vi "2012 Host Approach.vi"() -> ()   [LabVIEW 2013]
uses:
  <vilib>/rvi/interface/nirviOpenFPGA/nirviOpenFPGA.xnode
  <vilib>/rvi/interface/nirviReadWriteControl/nirviReadWriteControl.xnode
  <vilib>/rvi/interface/Simulation/niFpgaSimulationCallBeginRW.vi
  <vilib>/rvi/errors/niLvFpgaAdjustHostInterfaceError.vi
  <vilib>/rvi/interface/nirviCloseFPGA/nirviCloseFPGA.xnode
  <vilib>/FPGAPlugInAG/Dynamic/niLvFpga_Close_Dynamic.vi
  <vilib>/rvi/interface/nirviMethod/nirviMethod.xnode
  <vilib>/FPGAPlugInAG/Dynamic/niLvFpga_Run_Dynamic.vi
panel:
  in  "Automated Approach Start":bool
  out "FPGA Output Voltage":dbl(graph)
  in  "MCL Counter":i64
  in  "MCL Divisions":i32
  out "MCL Range Indicator":bool
  out "Host Counter Indicator":i64
  out "Digital Steps per Region":i32
  out "Host Counter Output":i32
  in  "Z Position MCL Fine":i32
  out "Host Z Position Indicator":i32
  out "Z Position Range Indicator":bool
  out "Z Fine Steps per Region":dbl
  out "Host Z Output":fxp<+/-,40,30>
  in  "Manual Approach Start":bool
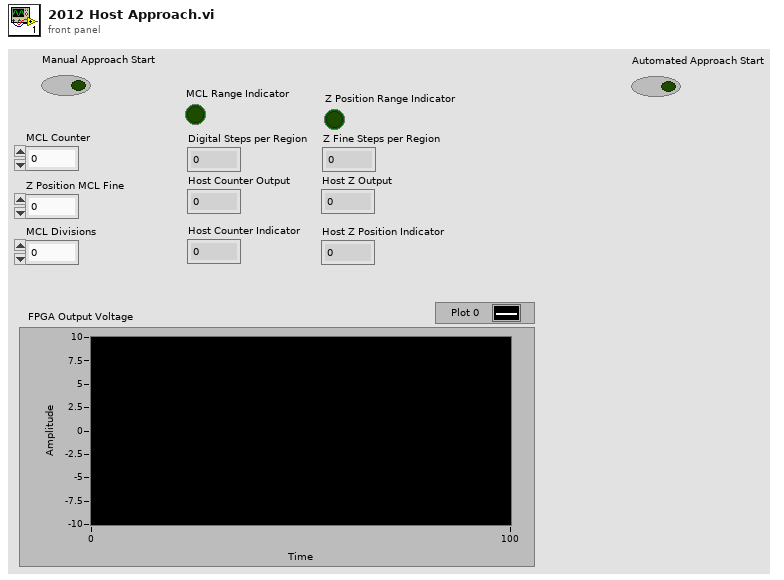
[diagram p1: front panel]
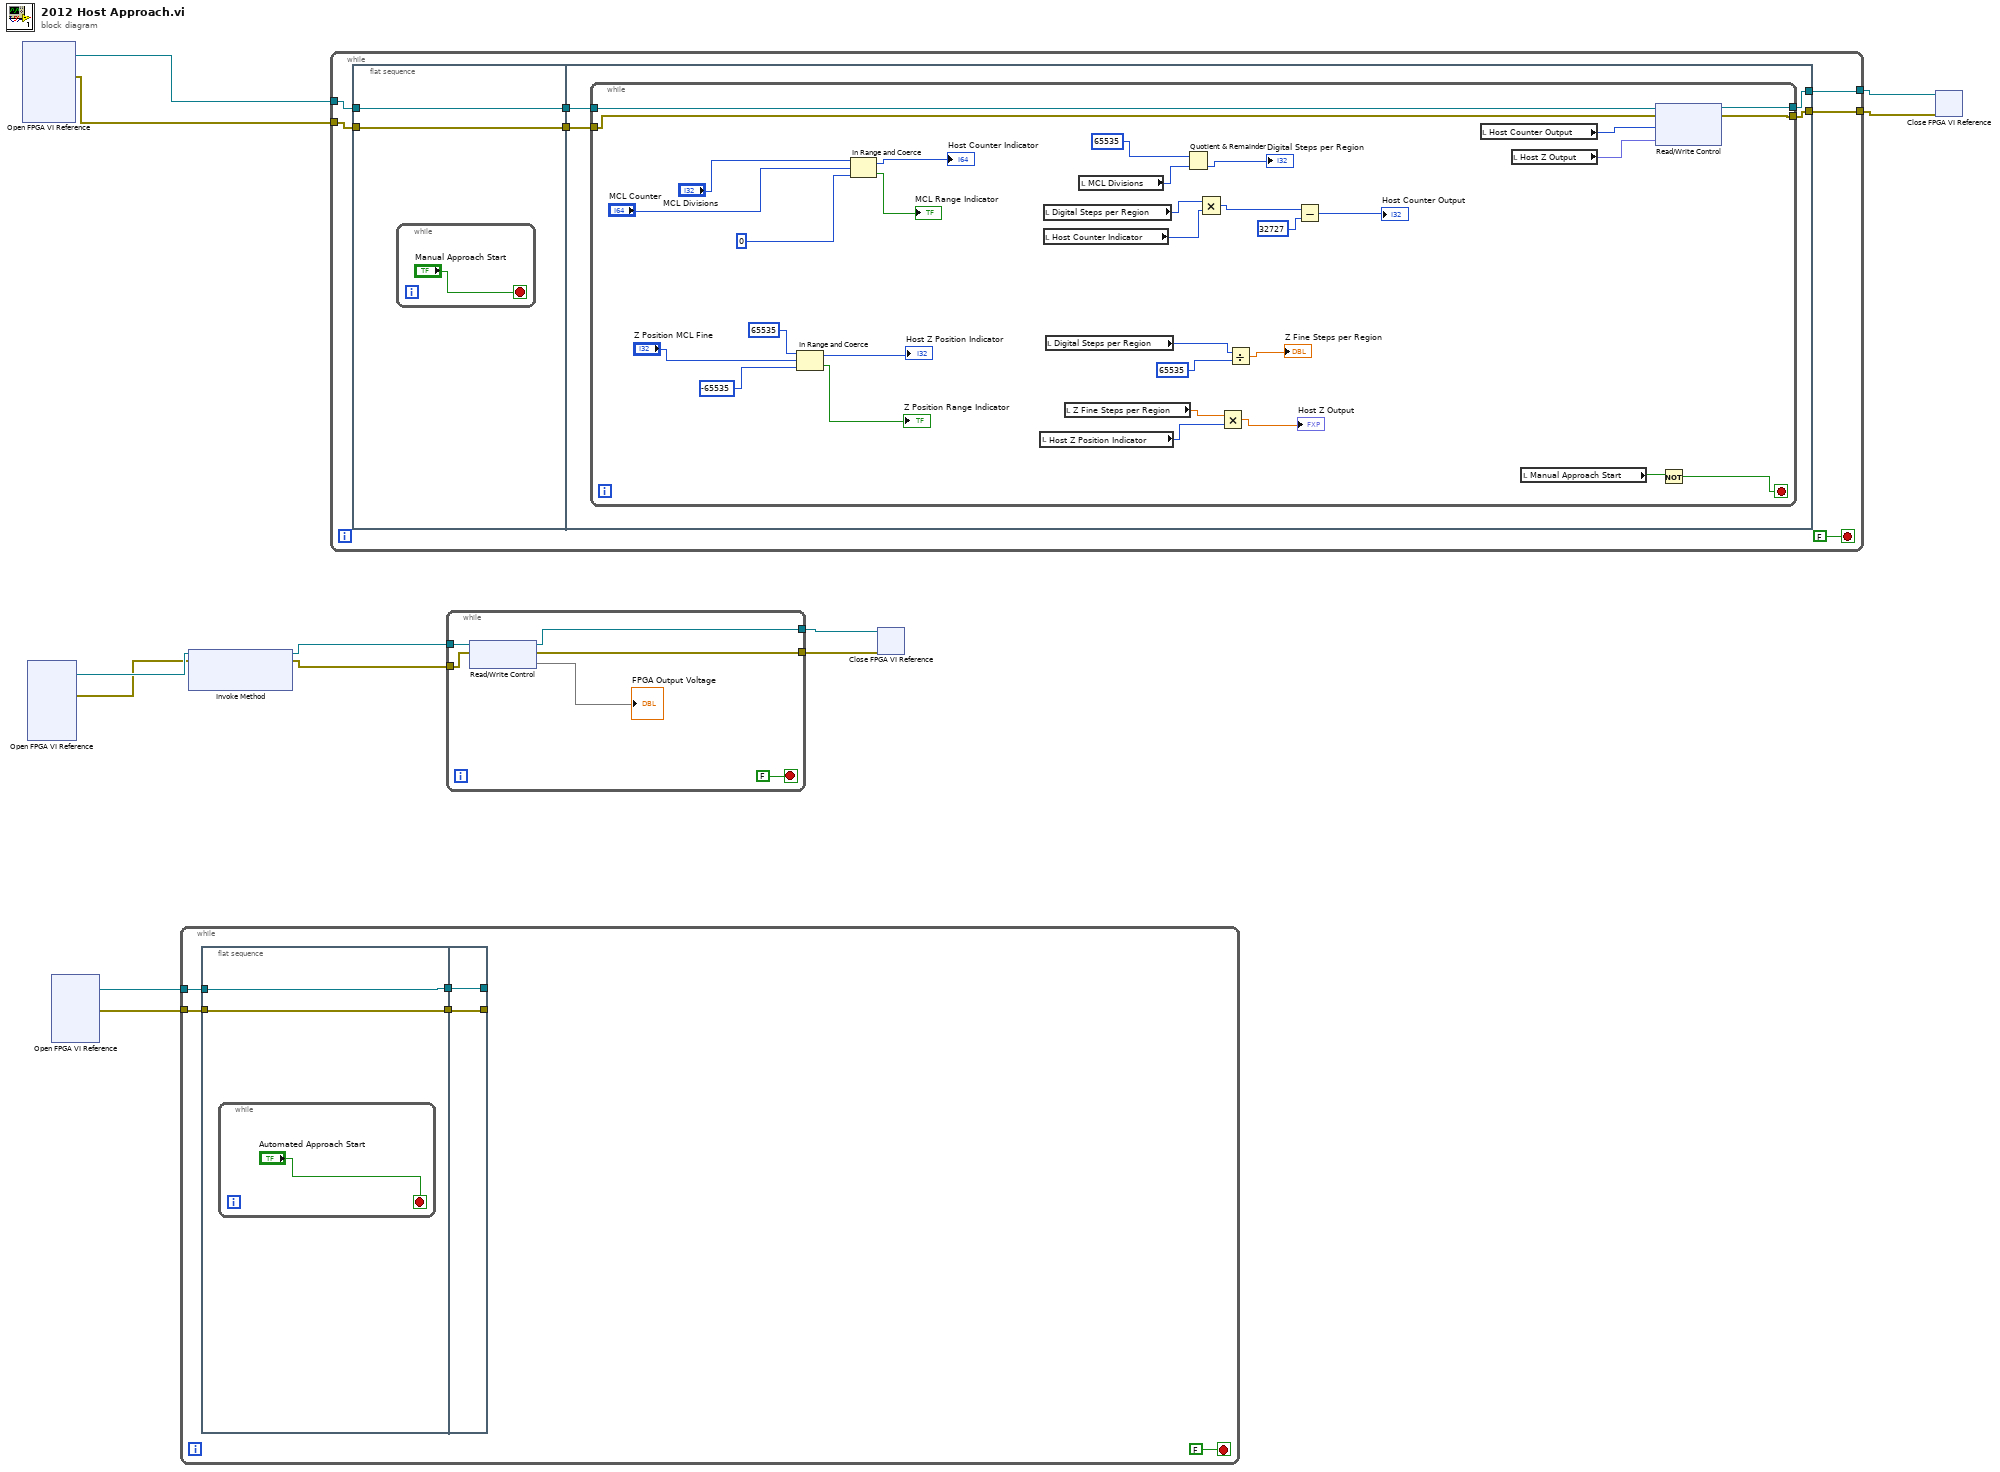
[diagram p0: block diagram]
diagram:
  n1 = xnode "Open FPGA VI Reference"() -> ("FPGA VI Reference Out"=w10:refnum<k20>, "error out"=w9:errorcluster)  [unwired: 2 in]
  n2 = xnode "Open FPGA VI Reference"() -> ("FPGA VI Reference Out"=w4:refnum<k20>, "error out"=w3:errorcluster)  [unwired: 2 in]
  n3 = xnode "Open FPGA VI Reference"() -> ("FPGA VI Reference Out"=w2:refnum<k20>, "error out"=w1:errorcluster)  [unwired: 2 in]
  n4 = while {
    tunnel: w2 -> [w16]
    tunnel: w1 -> [w15]
    stop <- FALSE stop-if-true
    n5 = flat-sequence {
      tunnel: w16 -> [w19]
      tunnel: w15 -> [w18]
      tunnel: [w19] -> w14
      tunnel: [w18] -> w13
      tunnel: [w21] -> _
      tunnel: [w22] -> _
      tunnel: w14 -> [w22]
      tunnel: w13 -> [w21]
      frame #0 {
        n6 = while {
          stop <- "Automated Approach Start" stop-if-true
        }
      }
      frame #1 {
      }
    }
  }
  n7 = xnode "Invoke Method"("FPGA VI Reference In"=w4, "error in"=w3) -> ("FPGA VI Reference Out"=w6:refnum<k20>, "error out"=w5:errorcluster)  [unwired: 1 in]
  n8 = while {
    tunnel: [w28] -> w12
    tunnel: [w27] -> w11
    tunnel: w10 -> [w25]
    tunnel: w9 -> [w23]
    stop <- FALSE stop-if-true
    n9 = flat-sequence {
      tunnel: [w31] -> w26
      tunnel: w25 -> [w31]
      tunnel: [w30] -> w24
      tunnel: w23 -> [w30]
      tunnel: [w34] -> w28
      tunnel: [w33] -> w27
      tunnel: w26 -> [w36]
      tunnel: w24 -> [w35]
      frame #0 {
        n10 = while {
          stop <- "Manual Approach Start" stop-if-true
        }
      }
      frame #1 {
        n11 = while {
          tunnel: w36 -> [w68]
          tunnel: w35 -> [w67]
          tunnel: [w66] -> w34
          tunnel: [w65] -> w33
          stop <- w63 stop-if-true
          n12 = In Range and Coerce(upper limit=65535, x="Z Position MCL Fine", lower limit=-65535) -> (coerced(x)=→"Host Z Position Indicator":i32, In Range?=→"Z Position Range Indicator":bool)
          n13 = In Range and Coerce(upper limit="MCL Divisions", x="MCL Counter", lower limit=0) -> (coerced(x)=→"Host Counter Indicator":i64, In Range?=→"MCL Range Indicator":bool)
          n14 = local read "Host Z Position Indicator"() -> (w39:i32)
          n15 = local read "Digital Steps per Region"() -> (w52:i32)
          n16 = local read "Host Counter Indicator"() -> (w51:i64)
          n17 = local read "Digital Steps per Region"() -> (w43:i32)
          n18 = local read "Z Fine Steps per Region"() -> (w40:dbl)
          n19 = local read "MCL Divisions"() -> (w56:i32)
          n20 = Quotient & Remainder(x=65535, y=w56) -> (floor(x/y)=→"Digital Steps per Region":i32)  [unwired: 1 out]
          n21 = Multiply(x=w52, y=w51) -> (x*y=w53:i64)
          n22 = Multiply(x=w40, y=w39) -> (x*y=→"Host Z Output":dbl)
          n23 = Divide(x=w43, y=65535) -> (x/y=→"Z Fine Steps per Region":dbl)
          n24 = Subtract(x=w53, y=32727) -> (x-y=→"Host Counter Output":i64)
          n25 = local read "Host Counter Output"() -> (w49:i32)
          n26 = local read "Host Z Output"() -> (w37:fxp<+/-,40,30>)
          n27 = local read "Manual Approach Start"() -> (w64:bool)
          n28 = xnode "Read/Write Control"("FPGA VI Reference In"=w68, "error in"=w67, "Unselected"=w49, "Unselected"=w37) -> ("FPGA VI Reference Out"=w66:refnum<k20>, "error out"=w65:errorcluster)
          n29 = Not(x=w64) -> (.not. x?=w63:bool)
        }
      }
    }
  }
  n30 = while {
    tunnel: w6 -> [w73]
    tunnel: w5 -> [w72]
    tunnel: [w71] -> w8
    tunnel: [w70] -> w7
    stop <- FALSE stop-if-true
    n31 = xnode "Read/Write Control"("FPGA VI Reference In"=w73, "error in"=w72) -> ("FPGA VI Reference Out"=w71:refnum<k20>, "error out"=w70:errorcluster, "Unselected"=→"FPGA Output Voltage")
  }
  n32 = xnode "Close FPGA VI Reference"("FPGA VI Reference In"=w8, "error in"=w7) -> ()  [unwired: 1 out]
  n33 = xnode "Close FPGA VI Reference"("FPGA VI Reference In"=w12, "error in"=w11) -> ()  [unwired: 1 out]
